vi "CRYGet DataView From QueueName.vi"(11 "DataView QueueName":string) -> (1 "DataView Idx out":i32, 2 "DataView out":T1, 3 "DataView Arrary Idx out":i32)   [LabVIEW 2013]
uses:
  Control/Graph Main Info Cluster.ctl
  Control/SplitterBar.ctl
  CRYNew View Global.vi
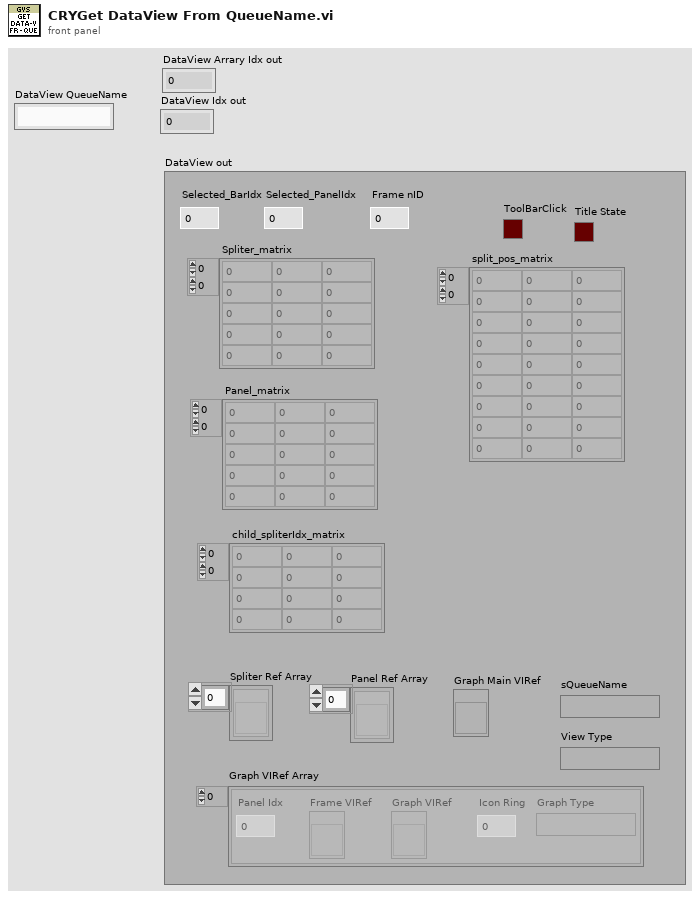
[diagram p1: front panel]
types:
  T1 = typedef "Graph Main Info Cluster.ctl" = cluster{"Selected_BarIdx":i32, "Selected_PanelIdx":i32, "Graph Main VIRef":refnum<vi>, "ToolBarClick":bool, "Spliter Ref Array":refnum<vi>[], "Panel Ref Array":refnum<vi>[], "Spliter_matrix":i32[][], "Panel_matrix":i32[][], "child_spliterIdx_matrix":i32[][], "split_pos_matrix":i32[][], "Title State":bool, "sQueueName":string, "Frame nID":i32, "Graph VIRef Array":cluster{"Graph VIRef":refnum<vi>, "Panel Idx":i32, "Frame VIRef":refnum<vi>, "Icon Ring":i32, "Graph Type":string}[], "View Type":string}
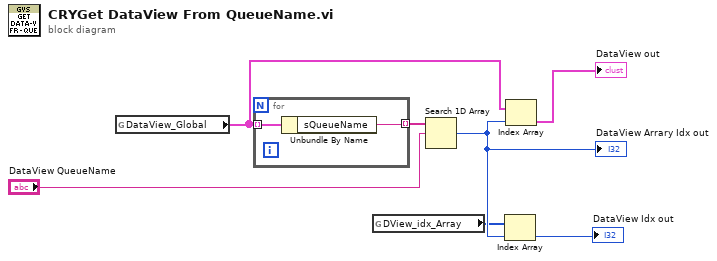
[diagram p0: block diagram]
diagram:
  n1 = global read "CRYNew View Global.vi" "DataView_Global"() -> (w5:T1[])
  n2 = for {
    tunnel: w5 -> [w9] mode=indexing
    tunnel: [w8] -> w7 mode=indexing
    n3 = Unbundle By Name(w9) -> ("sQueueName"=w8:string)
  }
  n4 = global read "CRYNew View Global.vi" "DView_idx_Array"() -> (w2:i32[])
  n5 = Search 1D Array(1D array=w7, element="DataView QueueName") -> (index of element=w3:i32)  [unwired: 1 in]
  "DataView Arrary Idx out" <- w3
  n6 = Index Array(array=w2, index=w3) -> (element=→"DataView Idx out":i32)
  n7 = Index Array(array=w5, index=w3) -> (element=→"DataView out":T1)
